vi "Hardware Device Get Info.vi"(8 "error in":errorcluster, 11 "NI PWM Output in":refnum<class "NI PWM Output.lvclass">) -> (0 "error out":errorcluster, 3 "NI PWM Output out":refnum<class "NI PWM Output.lvclass">)   [LabVIEW 2023, in "HardwareAbstractionLayer_LVOOP.lvlib" / "NI PWM Output.lvclass"]
doc: "This VI Device Physical Channel Read"
uses:
  NI PWM Output.lvclass
  NI PWM Output.lvclass/NI PWM Output.ctl
  <resource>/objmgr/daqmx.rc
  Teststand/Teststand.lvclass
panel:
  out "CO.PhysicalChans":tag[](array[tag])
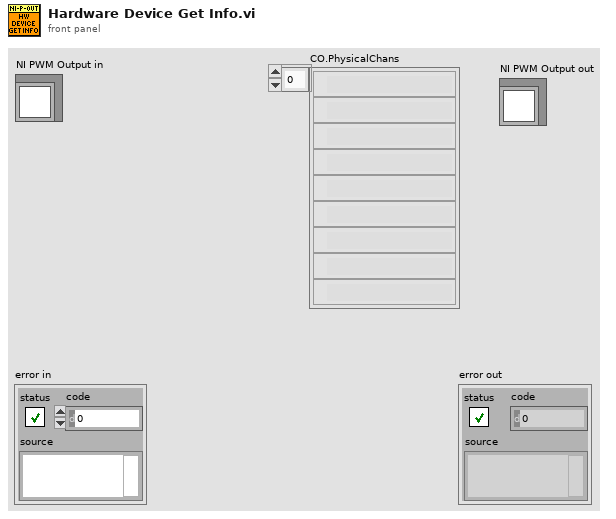
[diagram p1: front panel]
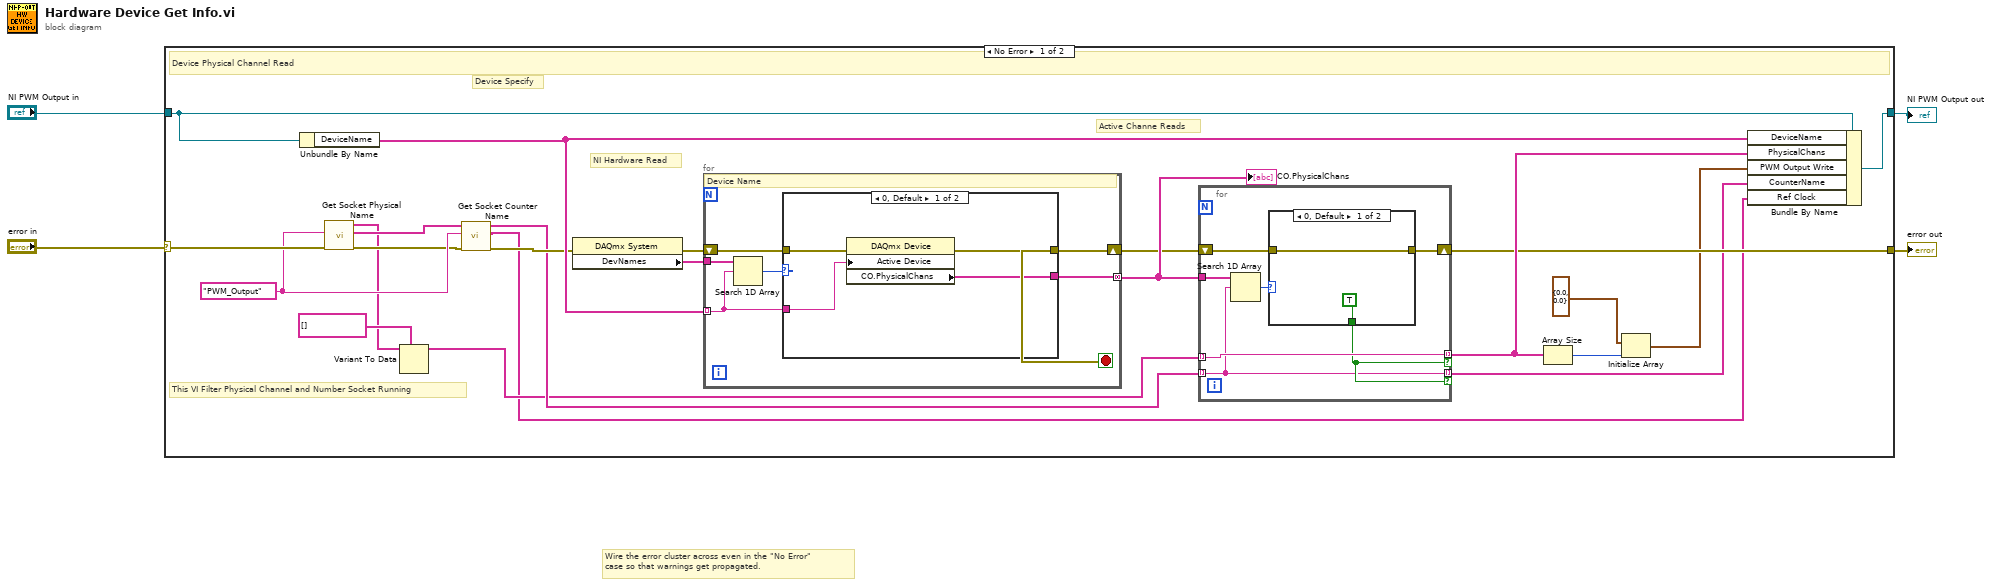
[diagram p0: block diagram]
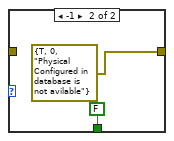
[diagram p2: hidden frame]
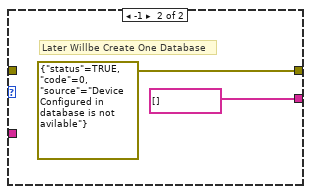
[diagram p3: hidden frame]
diagram:
  # "Wire the error cluster across even in the \"No Error\"\ncase so that warnings get propagated."
  n1 = case shown="No Error" "error in" {
    selector: "error in" -> [w18 w52]
    tunnel: [w17 w52] -> w3
    tunnel: [w22 w51] -> w1
    tunnel: "NI PWM Output in" -> [w21 w51]
    frame No Error {
      w13 = "PWM_Output" ("ChannelType")
      # "This VI Filter Physical Channel and Number Socket Running"
      # "Active Channe Reads"
      # "Device Specify"
      # "NI Hardware Read"
      # "Device Physical Channel Read"
      n2 = Unbundle By Name(w21) -> ("DeviceName"=w27:tag[])
      n3 = call "Get Socket Physical Name.vi"("error In"=w18, "ChannelType"=w13) -> ("error out"=w12:errorcluster, "Physical Channel"=w14:tag[], "Physical String"=w8:string[])  [unwired: 7 in]
      n4 = Variant To Data(type=tag[] [] ("CounterName"), Variant=w8) -> (data=w7:tag[])  [unwired: 1 in, 1 out]
      n5 = call "Get Socket Counter Name.vi"("error In"=w12, "ChannelType"=w13, "Physical Channel"=w14) -> ("error out"=w11:errorcluster, "ReferenceClock"=w5:tag[], "CounterName"=w10:tag[])  [unwired: 6 in]
      n6 = property class="DAQmx System"(error in=w11) -> (error out=w25:errorcluster, "DevNames"=w26:tag[])  [unwired: 1 in, 1 out]
      n7 = for {
        tunnel: w27 -> [w41] mode=indexing
        tunnel: w26 -> [w42]
        tunnel: [w40] -> w24 mode=concatenating
        shift-right: [w39] -> w23
        shift-left: w25 -> [w43]
        stop <- w39 stop-if-true
        # "Device Name"
        n8 = Search 1D Array(1D array=w42, element=w41) -> (index of element=w44:i32)  [unwired: 1 in]
        n9 = case shown="0, Default" w44 {
          tunnel: w43 -> [w46 _]
          tunnel: [w45 errorcluster {"status"=TRUE, "code"=0, "source"="Device  Configured in database is not avilable"} ("error out")] -> w39
          tunnel: w41 -> [w48 _]
          tunnel: [w47 tag[] [] ("AI.PhysicalChans")] -> w40
          frame 0, Default {
            n10 = property class="DAQmx Device"(error in=w46, "Active Device"=w48) -> (error out=w45:errorcluster, "CO.PhysicalChans"=w47:tag[])  [unwired: 1 in, 1 out]
          }
          frame -1 {
            # "Later Willbe Create One Database"
          }
        }
      }
      "CO.PhysicalChans" <- w24
      n11 = for {
        tunnel: w24 -> [w34]
        tunnel: w7 -> [w30] mode=indexing
        shift-right: [w31] -> w17
        shift-left: w23 -> [w32]
        tunnel: [w30] -> w20 mode=indexing if=w29
        tunnel: w10 -> [w28] mode=indexing
        tunnel: [w28] -> w6 mode=indexing if=w29
        n12 = Search 1D Array(1D array=w34, element=w28) -> (index of element=w33:i32)  [unwired: 1 in]
        n13 = case shown="0, Default" w33 {
          tunnel: w32 -> [w36 _]
          tunnel: [w36 errorcluster {"status"=TRUE, "code"=0, "source"="Physical Configured in database is not avilable"} ("error out")] -> w31
          tunnel: [TRUE FALSE] -> w29
          frame 0, Default {
          }
          frame -1 {
          }
        }
      }
      n14 = Array Size(array=w20) -> (size(s)=w19:i32)
      n15 = Initialize Array(cluster{"duty cycle":dbl, "frequency":dbl} {"duty cycle"=0.0, "frequency"=0.0} ("values"), w19) -> (w16:cluster{"duty cycle":dbl, "frequency":dbl}[])
      n16 = Bundle By Name(cluster=w21, "DeviceName"=w27, "PhysicalChans"=w20, "PWM Output Write"=w16, "CounterName"=w6, "Ref Clock"=w5) -> (w22:refnum<class "NI PWM Output.lvclass">)
    }
    frame Error {
    }
  }
  "error out" <- w3
  "NI PWM Output out" <- w1
